vi "ICR_Timer_Start_Async.vi"(0 "Seconds":dbl=5.0 format="%#_13g", 1 "Last Seconds":dbl=5.0 format="%#_13g", 2 "Refnum Ch":refnum<vi>, 3 "error in (no error)":errorcluster) -> (10 "error out":errorcluster)   [LabVIEW 2020]
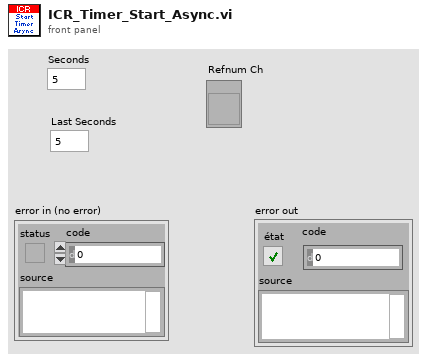
[diagram p1: front panel]
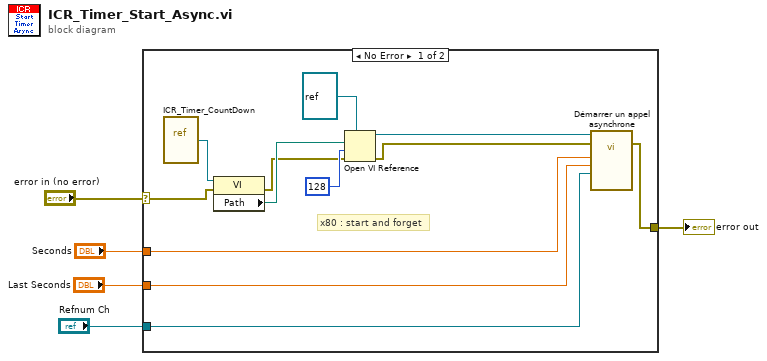
[diagram p0: block diagram]
diagram:
  n1 = case shown="No Error" "error in (no error)" {
    selector: "error in (no error)" -> [w14 w18]
    tunnel: [w15 w18] -> w4
    tunnel: "Seconds" -> [w12 _]
    tunnel: "Refnum Ch" -> [w6 _]
    tunnel: "Last Seconds" -> [w7 _]
    frame No Error {
      # "x80 : start and forget"
      n2 = vi-ref "ICR_Timer_CountDown.vi"() -> (w10:refnum<vi>)
      n3 = property class="VI"(reference=w10, error in=w14) -> (error out=w13:errorcluster, "Path"=w16:path)  [unwired: 1 out]
      n4 = Open VI Reference(type specifier VI Refnum (for type only)=refnum<vi> refnum ("spécificateur de type du refnum de VI (pour type seulement)"), vi path=w16, options=128, error in (no error)=w13) -> (vi reference=w8:refnum<vi>, error out=w11:errorcluster)  [unwired: 2 in]
      n5 = call-by-ref "Démarrer un appel asynchrone"(reference=w8, error in=w11, "Seconds"=w12, "Last Seconds"=w7, "Refnum Ch"=w6) -> (error out=w15:errorcluster)  [unwired: 8 in, 1 out]
    }
    frame Error {
    }
  }
  "error out" <- w4
